vi "Get Server Internal UEs.vi"(11 "OOP Server in":refnum<class "OCV.lvclass">) -> (2 "Server Internal UEs":T1, 3 "OOP Server out":refnum<class "OCV.lvclass">)   [LabVIEW 2019, in "OCV.lvlib" / "OCV.lvclass"]
uses:
  OCV.lvclass
  typeDefs/Server Internal UEs.ctl
  typeDefs/Server Internal Message UE.ctl
  typeDefs/Server Internal Message.ctl
  OCV.lvclass/OCV.ctl
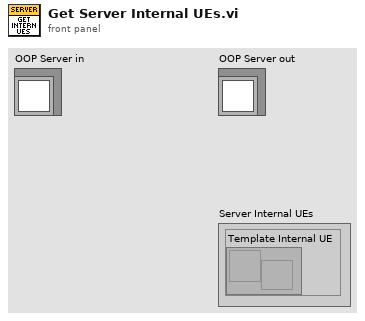
[diagram p1: front panel]
types:
  T1 = typedef "OCV.lvlib/OCV.lvclass/Server Internal UEs.ctl" = cluster{"Template Internal UE":T2}
  T2 = typedef "OCV.lvlib/OCV.lvclass/Server Internal Message UE.ctl" = refnum<user-event>
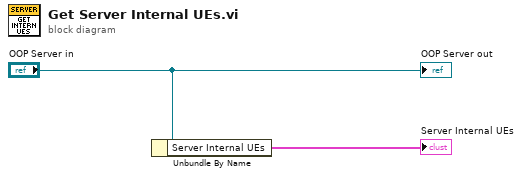
[diagram p0: block diagram]
diagram:
  n1 = Unbundle By Name("OOP Server in") -> ("Server Internal UEs"=→"Server Internal UEs":T1)
  "OOP Server out" <- "OOP Server in"
